vi "_Parse SEM Segment Result.vi"(8 "error in (no error)":errorcluster, 10 "Input String":string, 11 "VISA resource name":refnum<visa-resource-name>) -> (0 "error out":errorcluster, 1 "SEM Results":cluster{"OBW":dbl, "TX Power":dbl} {"TX Power" format="%^.3e"; "OBW" format="%^.3e"}, 2 "Reliability Results":T1, 3 "VISA resource name out":refnum<visa-resource-name>, 5 "Out Of Tolerance":dbl format="%^.3e", 7 "Statistic Expired":i32)   [LabVIEW 2015, in "Rohde&Schwarz CMXP NR FR2 Measurement.lvlib"]
uses:
  <instrlib>/Rohde&Schwarz CMXP NR FR2 Measurement/Rohde&Schwarz CMXP NR FR2 Measurement.lvlib
  <instrlib>/Rohde&Schwarz CMXP NR FR2 Measurement/Private/rsidr_core.llb/rsidr_core.lvlib
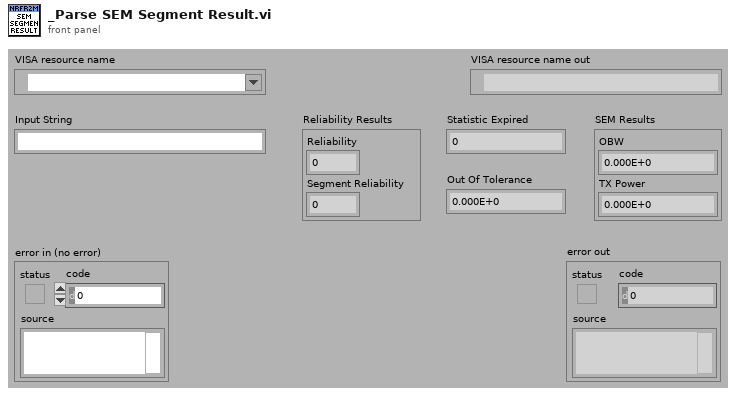
[diagram p1: front panel]
types:
  T1 = cluster{"Reliability":i32, "Segment Reliability":i32}
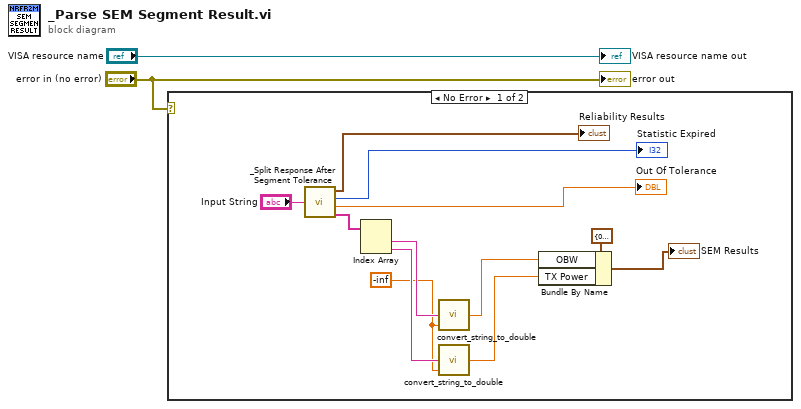
[diagram p0: block diagram]
diagram:
  n1 = case shown="No Error" "error in (no error)" {
    frame No Error {
      w7 = -inf
      n2 = call <instrlib>:"_Split Response After Segment Tolerance.vi"("Input String"="Input String") -> ("Reliability Results"=→"Reliability Results":T1, "Statistic Expired"=→"Statistic Expired":i32, "Out Of Tolerance"=→"Out Of Tolerance":dbl, "Response out"=w12:string[])
      n3 = Index Array(array=w12) -> (element #1=w11:string, element #2=w10:string)  [unwired: 2 in]
      n4 = call <instrlib>:"convert_string_to_double.vi"("default (0)"=w7, "String in"=w11) -> ("double value out"=w14:dbl)  [unwired: 3 in]
      n5 = call <instrlib>:"convert_string_to_double.vi"("default (0)"=w7, "String in"=w10) -> ("double value out"=w9:dbl)  [unwired: 3 in]
      n6 = Bundle By Name(cluster=cluster{"OBW":dbl, "TX Power":dbl} {"OBW"=0.0, "TX Power"=0.0} ("SEM Results"), "OBW"=w14, "TX Power"=w9) -> (→"SEM Results":cluster{"OBW":dbl, "TX Power":dbl})
    }
    frame Error {
    }
  }
  "error out" <- "error in (no error)"
  "VISA resource name out" <- "VISA resource name"
